vi "Escape URL Component.vi"(11 "URL component in":string) -> (3 "URL component out":string)   [LabVIEW 2015, in "NI_Azure_Core.lvlib"]
uses:
  NI_Azure_Core.lvlib
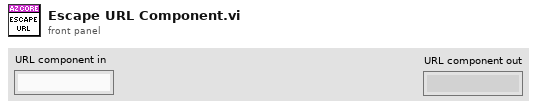
[diagram p1: front panel]
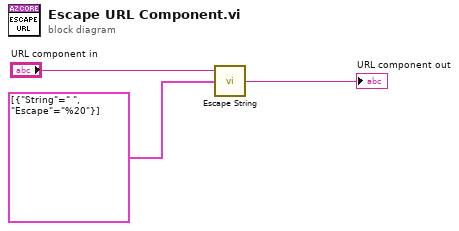
[diagram p0: block diagram]
diagram:
  n1 = call <vilib>:"Escape String.vi"("Escapes"=cluster{"String":string, "Escape":string}[] [{"String"=" ", "Escape"="%20"}], "String in"="URL component in") -> ("String out"=→"URL component out":string)  [unwired: 1 in]
